vi "Subvi counter pixels U16.vi"(4 "Reset":bool, 9 "Pixel clock":bool) -> (1 "Pixel count":u16)   [LabVIEW 2017]
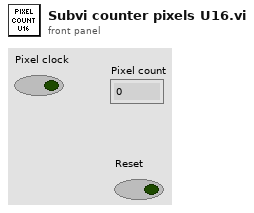
[diagram p1: front panel]
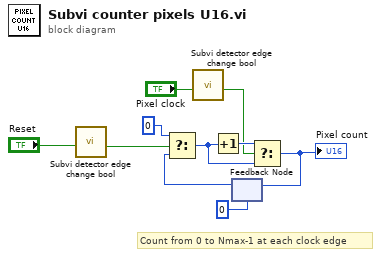
[diagram p0: block diagram]
diagram:
  # "Count from 0 to Nmax-1 at each clock edge"
  n1 = call "Subvi detector edge change bool.vi"("Input"="Reset") -> ("Output"=w2:bool)  [unwired: 8 in]
  n2 = call "Subvi detector edge change bool.vi"("Input"="Pixel clock") -> ("Output"=w3:bool)  [unwired: 8 in]
  n3 = feedback #1(u16 0) -> (w5:u16)
  n4 = Select(t=u16 0, s=w2, f=w5) -> (s? t:f=w6:u16)
  n5 = Increment(x=w6) -> (x+1=w7:u16)
  n6 = Select(t=w7, s=w3, f=w6) -> (s? t:f=w9:u16)
  "Pixel count" <- w9
  n7 = feedback-in #1(w9) -> ()
